vi "test_serialize_deserialize.vi"   [LabVIEW 2020, in "LIN Frame Array.lvlib"]
doc: "Version 0.1"
uses:
  <vilib>/ADAS Record/CustomDataTypes/LIN Frame Array/LIN Frame Array.lvlib
  <vilib>/addons/_JKI Toolkits/Caraya/classes/Test/Test.lvclass
  <vilib>/addons/_JKI Toolkits/Caraya/classes/Assert/Assert.lvclass
  <vilib>/ADAS Record/CustomDataTypes/LIN Frame Array/Process Data.ctl
  <vilib>/ADAS Record/CustomDataTypes/LIN Frame Array/Serialize Data.vi
  <vilib>/ADAS Record/CustomDataTypes/LIN Frame Array/Deserialize Data.vi
  <vilib>/ADAS Record/CustomDataTypes/LIN Frame Array/LIN Frame.ctl
types:
  T1 = typedef "LIN Frame Array.lvlib/LIN Frame.ctl" = cluster{"timestamp":timestamp, "payload":u8[], "identifier":u32, "type":u8, "event ID":u8, "event slot?":bool, "echo?":bool}
  T2 = typedef "LIN Frame Array.lvlib/Process Data.ctl" = cluster{"Timestamp":timestamp, "Bus Channel":u16, "LIN Frame Array":T1[]}
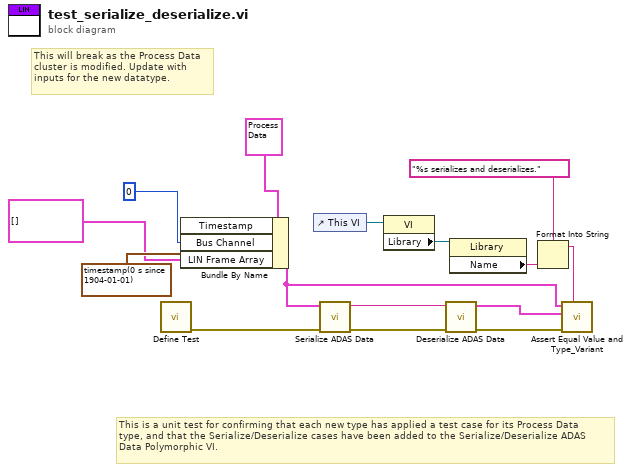
[diagram p0: block diagram]
diagram:
  # "This will break as the Process Data\ncluster is modified. Update with\ninputs for the new datatype."
  # "This is a unit test for confirming that each new type has applied a test case for its Process Data\ntype, and that the Serialize/Deserialize cases have been added to the Serialize/Deserialize ADAS\nData Polymorphic VI."
  n1 = call <vilib>:"Define Test.vi"() -> ("error out"=w10:errorcluster)  [unwired: 11 in]
  n2 = Bundle By Name "Bundle By Name"(cluster=T2 {"Timestamp"=timestamp(0 s since 1904-01-01), "Bus Channel"=0, "LIN Frame Array"=[]} ("Process Data in"), "Timestamp"=timestamp(0 s since 1904-01-01), "Bus Channel"=u16 0, "LIN Frame Array"=T1[] []) -> (w4:T2)
  n3 = control-ref of="This VI"() -> (w15:refnum<vi>)
  n4 = call-poly <vilib>:"Serialize ADAS Data.vi"("error in (no error)"=w10, "Process Data"=w4) -> ("error out"=w9:errorcluster, "Flat Data out"=w8:string)  [unwired: 8 in]
  n5 = property class="VI"(reference=w15) -> ("Library"=w14:refnum<vi>)  [unwired: 1 in, 2 out]
  n6 = call-poly <vilib>:"Deserialize ADAS Data.vi"("error in (no error)"=w9, "Flat Data in"=w8) -> ("error out"=w6:errorcluster, "Process Data out"=w7:T2)  [unwired: 8 in]
  n7 = property class="Library"(reference=w14) -> ("Name"=w12:string)  [unwired: 1 in, 2 out]
  n8 = Format Into String(format string="%s serializes and deserializes.", w12) -> (resulting string=w11:string)  [unwired: 2 in, 1 out]
  n9 = call <vilib>:"Assert Equal Value and Type_Variant.vi"("Label"=w11, "error in (no error)"=w6, "Y"=w7, "X"=w4) -> ()  [unwired: 7 in, 1 out]
